vi "dB to Multiplier.vi"(11 "Attenuation":dbl=128.0) -> (3 "Multiplier":dbl)   [LabVIEW 2015]
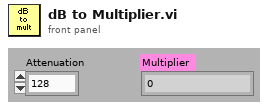
[diagram p1: front panel]
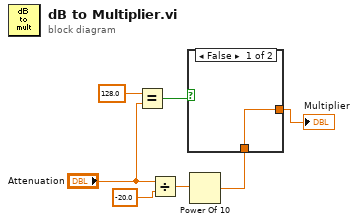
[diagram p0: block diagram]
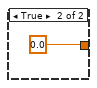
[diagram p2: hidden frame]
diagram:
  n1 = Equal?(x=128.0, y="Attenuation") -> (x = y?=w3:bool)
  n2 = Divide(x="Attenuation", y=-20.0) -> (x/y=w6:dbl)
  n3 = Power Of 10(x=w6) -> (10^x=w2:dbl)
  n4 = case shown="False" w3 {
    tunnel: [w8 0.0] -> w1
    tunnel: w2 -> [w8 _]
    frame False {
    }
    frame True {
    }
  }
  "Multiplier" <- w1
